vi "libssh2_channel_forward_listen_ex.vi"(7 "queue_maxsize":i32, 8 "error in (no error)":errorcluster, 9 "port in":i32, 10 "host":string, 11 "session":T2) -> (0 "error out":errorcluster, 1 "port out":i32, 3 "listener":T1)   [LabVIEW 2013, in "libssh2.lvlib"]
doc: "Create a listening channel for inbound TCP connections on a specific address and port on the SSH server. New connections are queued until accepted with <B>libssh2_channel_forward_accept</B>."
uses:
  libssh2.lvlib
  Session Refnum.ctl
  Listener Refnum.ctl
  Not A Session.vi
  <vilib>/Utility/error.llb/Error Cluster From Error Code.vi
  Global Settings.vi
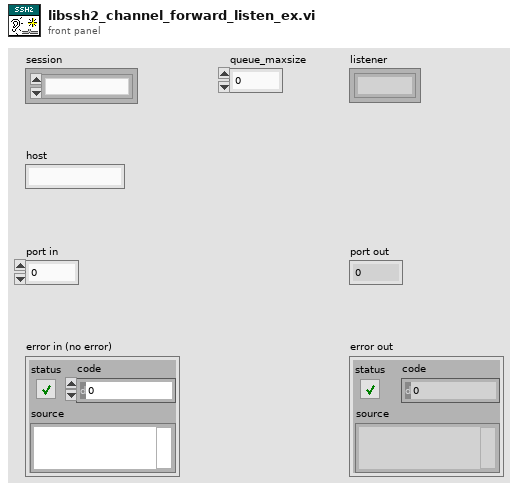
[diagram p1: front panel]
types:
  T1 = typedef "libssh2.lvlib/Listener Refnum.ctl" = refnum<k1>
  T2 = typedef "libssh2.lvlib/Session Refnum.ctl" = refnum<k1>
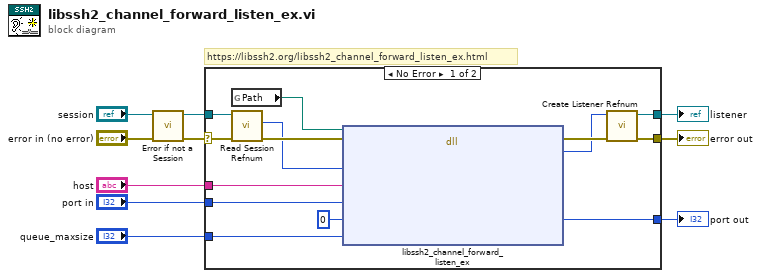
[diagram p0: block diagram]
diagram:
  # "https://libssh2.org/libssh2_channel_forward_listen_ex.html"
  n1 = call "Error if not a Session.vi"("error in (no error)"="error in (no error)", "session"="session") -> ("error out"=w3:errorcluster, "session out"=w1:T2)  [unwired: 8 in]
  n2 = case shown="No Error" w3 {
    selector: w3 -> [w12 w25]
    tunnel: "host" -> [w23 _]
    tunnel: "port in" -> [w22 _]
    tunnel: "queue_maxsize" -> [w21 _]
    tunnel: [w19 _] -> w7
    tunnel: w1 -> [w17 _]
    tunnel: [w15 w25] -> w6
    tunnel: [w13 _] -> w5
    frame No Error {
      n3 = global read "Global Settings.vi" "Path"() -> (w11:path)
      n4 = call "Read Session Refnum.vi"("error in (no error)"=w12, "session"=w17) -> ("error out"=w18:errorcluster, "LIBSSH2_SESSION*"=w16:u64)  [unwired: 5 in, 3 out]
      n5 = dll-call lib="?" fn="libssh2_channel_forward_listen_ex"(path in=w11, error in=w18, "session"=w16, "host"=w23, "port"=w22, "bound_port"=0, "queue_maxsize"=w21) -> (error out=w24:errorcluster, "return value"=w14:u64, "bound_port"=w19:i32)  [unwired: 5 in, 1 out]
      n6 = call "Create Listener Refnum.vi"("error in (no error)"=w24, "LIBSSH2_LISTENER*"=w14) -> ("error out"=w15:errorcluster, "listener"=w13:T1)  [unwired: 8 in]
    }
    frame Error {
    }
  }
  "error out" <- w6
  "port out" <- w7
  "listener" <- w5
